vi "Test.vi"   [LabVIEW 2019]
doc: "This VI is called when test mode begins, and will automatically be terminated when it ends. You can add manual or automatic tests and invoke them from the dashboard."
uses:
  <vilib>/Rock Robotics/WPI/Ultrasonic/WPI_SonarSRF04DigitalRefNum Registry Get.vi
  <vilib>/Rock Robotics/WPI/Ultrasonic/WPI_SonarSRF04DigitalGetRange.vi
  <vilib>/Rock Robotics/WPI/Ultrasonic/WPI_UltrasonicRangeUnits.ctl
types:
  T1 = typedef "WPI_UltrasonicRangeUnits.ctl" = enum16{"inches", "mm"}
  T2 = typedef "WPI_UltrasonicDeviceRef.ctl" = cluster{"DevStatus":errorcluster, "Ping Channel":T3, "Echo Channel":T3, "CntIndex":T4}
  T3 = typedef "FPGA_DIOChannel.ctl" = enum8{"DIO 0", "DIO 1", "DIO 2", "DIO 3", "DIO 4", "DIO 5", "DIO 6", "DIO 7", "DIO 8", "DIO 9", "DIO MXP 0", "DIO MXP 1", "DIO MXP 2", "DIO MXP 3", "DIO MXP 4", "DIO MXP 5", "DIO MXP 6", "DIO MXP 7", "DIO MXP 8", "DIO MXP 9", "DIO MXP 10", "DIO MXP 11", "DIO MXP 12", "DIO MXP 13", "DIO MXP 14", "DIO MXP 15", "SPI Port CS1", "SPI Port CS2", "SPI Port CS3", "SPI Port MISO", "SPI Port MOSI", "Invalid"}
  T4 = typedef "FPGA_CounterCtrSystemIndex.ctl" = enum8{"Ctr 0", "Ctr 1", "Ctr 2", "Ctr 3", "Ctr 4", "Ctr 5", "Ctr 6", "Ctr 7", "Invalid"}
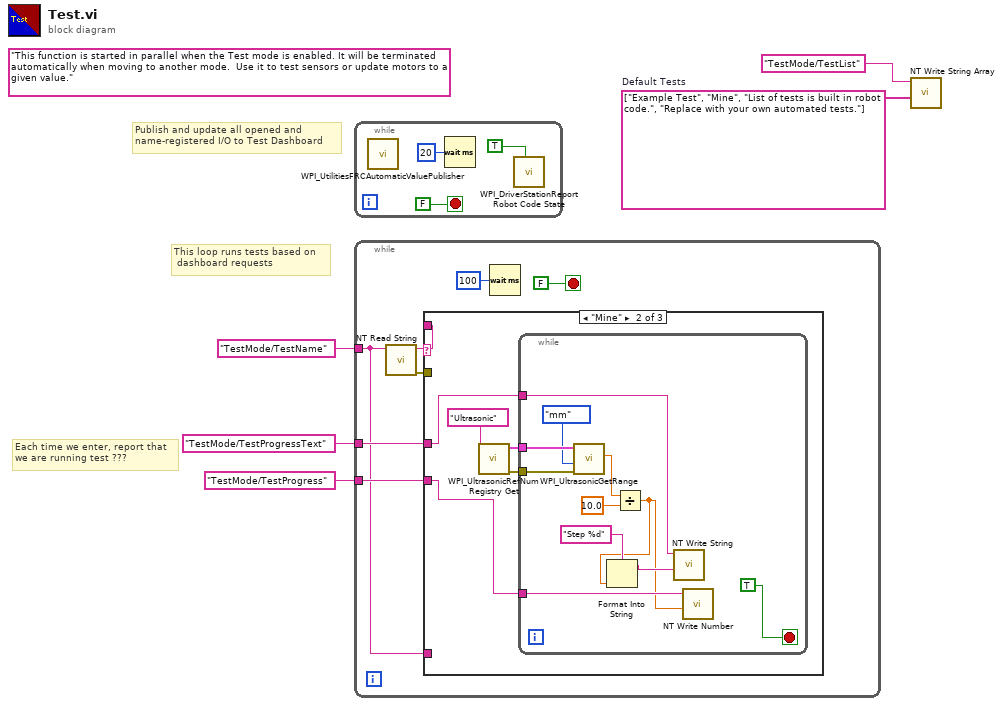
[diagram p0: block diagram]
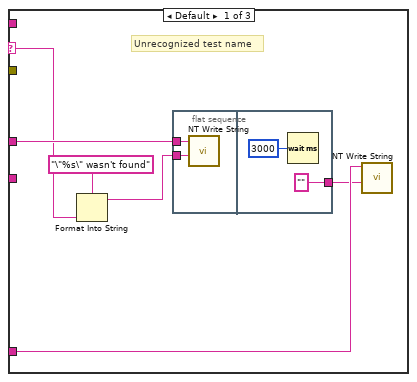
[diagram p2: hidden frame]
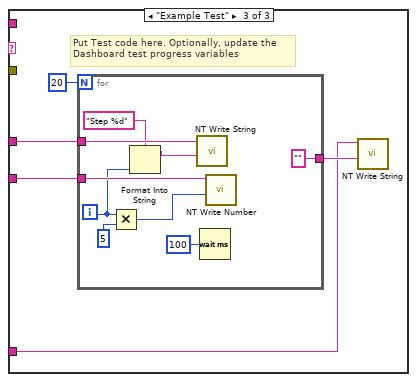
[diagram p3: hidden frame]
diagram:
  w2 = string[] ["Example Test", "Mine", "List of tests is built in robot code.", "Replace with your own automated tests."]  # Default Tests
  (unwired) "This function is started in parallel when the Test mode is enabled. It will be terminated automatically when moving to another mode.  Use it to test sensors or update motors to a given value."
  # "This loop runs tests based on \n dashboard requests"
  # "Publish and update all opened and\nname-registered I/O to Test Dashboard"
  # "Each time we enter, report that\nwe are running test ???"
  n1 = while {
    stop <- FALSE stop-if-true
    n2 = call <vilib>:"WPI_UtilitiesFRCAutomaticValuePublisher.vi"() -> ()  [unwired: 12 in]
    n3 = Wait (ms)(milliseconds to wait=u32 20) -> ()  [unwired: 1 out]
    n4 = call <vilib>:"WPI_DriverStationReport Robot Code State.vi"("Test"=TRUE ("Autonomous")) -> ()  [unwired: 10 in, 1 out]
  }
  n5 = while {
    tunnel: "TestMode/TestName" ("Name") -> [w10]
    tunnel: "TestMode/TestProgressText" ("Name") -> [w13]
    tunnel: "TestMode/TestProgress" ("Name") -> [w12]
    stop <- FALSE stop-if-true
    n6 = call <vilib>:"NT Read String.vi"("Name"=w10) -> ("error out"=w9:errorcluster, "String"=w11:string)  [unwired: 9 in]
    n7 = case shown="\"Mine\"" w11 {
      selector: w11 -> [w20 _ _]
      tunnel: w10 -> [w17 _ w42]
      tunnel: w13 -> [w21 w26 w45]
      tunnel: w12 -> [_ w27 w46]
      tunnel: w11 -> [_ _ _]
      tunnel: w9 -> [_ _ _]
      frame Default {
        # "Unrecognized test name"
        n8 = Format Into String(format string="\"%s\" wasn't found" ("Name"), w20) -> (resulting string=w19:string)  [unwired: 2 in, 1 out]
        n9 = flat-sequence {
          tunnel: w21 -> [w22]
          tunnel: w19 -> [w23]
          tunnel: ["" ("Name")] -> w16
          frame #0 {
            n10 = call <vilib>:"NT Write String.vi"("String"=w23, "Name"=w22) -> ()  [unwired: 9 in, 1 out]
          }
          frame #1 {
            n11 = Wait (ms)(milliseconds to wait=u32 3000) -> ()  [unwired: 1 out]
          }
        }
        n12 = call <vilib>:"NT Write String.vi"("String"=w16, "Name"=w17) -> ()  [unwired: 9 in, 1 out]
      }
      frame "Mine" {
        n13 = call-poly <vilib>:"WPI_UltrasonicRefNum Registry Get.vi"("refnum name"="Ultrasonic") -> ("error out"=w28:errorcluster, "SonarSRF04DevRef"=w29:T2)  [unwired: 9 in]
        n14 = while {
          tunnel: w29 -> [w41]
          tunnel: w28 -> [w40]
          tunnel: w27 -> [w34]
          tunnel: w26 -> [w33]
          stop <- TRUE stop-if-true
          n15 = call-poly <vilib>:"WPI_UltrasonicGetRange.vi"("error in (no error)"=w40, "Range Units"=WPI_UltrasonicRangeUnits."mm", "SonarSRF04DevRef"=w41) -> ("Distance"=w38:dbl)  [unwired: 6 in, 2 out]
          n16 = Divide(x=w38, y=10.0) -> (x/y=w32:dbl)
          n17 = Format Into String(format string="Step %d", w32) -> (resulting string=w35:string)  [unwired: 2 in, 1 out]
          n18 = call <vilib>:"NT Write String.vi"("String"=w35, "Name"=w33) -> ()  [unwired: 9 in, 1 out]
          n19 = call <vilib>:"NT Write Number.vi"("Numeric"=w32, "Name"=w34) -> ()  [unwired: 9 in, 1 out]
        }
      }
      frame "Example Test" {
        # "Put Test code here. Optionally, update the\nDashboard test progress variables"
        n20 = for {
          N: 20 -> [_]
          tunnel: w46 -> [w55]
          tunnel: w45 -> [w53]
          tunnel: ["" ("String")] -> w43
          i -> [w50]
          n21 = Multiply(x=w50, y=u32 5 ("milliseconds to wait")) -> (x*y=w51:u32)
          n22 = Format Into String(format string="Step %d", w50) -> (resulting string=w48:string)  [unwired: 2 in, 1 out]
          n23 = call <vilib>:"NT Write String.vi"("String"=w48, "Name"=w53) -> ()  [unwired: 9 in, 1 out]
          n24 = Wait (ms)(milliseconds to wait=u32 100) -> ()  [unwired: 1 out]
          n25 = call <vilib>:"NT Write Number.vi"("Numeric"=w51, "Name"=w55) -> ()  [unwired: 9 in, 1 out]
        }
        n26 = call <vilib>:"NT Write String.vi"("String"=w43, "Name"=w42) -> ()  [unwired: 9 in, 1 out]
      }
    }
    n27 = Wait (ms)(milliseconds to wait=u32 100) -> ()  [unwired: 1 out]
  }
  n28 = call <vilib>:"NT Write String Array.vi"("String Array"=w2, "Name"="TestMode/TestList") -> ()  [unwired: 9 in, 1 out]
